vi "Set BackColor.vi"(8 "error in":errorcluster, 10 "Color":T1, 11 "View in":refnum<class "Cell View.lvclass">) -> (0 "error out":errorcluster, 3 "View out":refnum<class "Cell View.lvclass">)   [LabVIEW 2023, in "SourceGrid.lvlib" / "Cell View.lvclass"]
uses:
  Cell View.lvclass
  Cell View.lvclass/Cell View.ctl
  D:/git/Sourcegrid-LabVIEW/dll/SourceGrid.dll
  dll/SourceGrid.dll
  Color/Color.lvclass
  System.Drawing.Color.ctl
  SourceGrid.lvlib
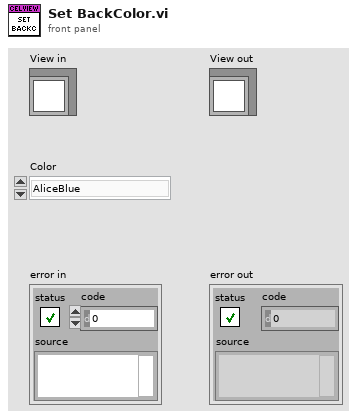
[diagram p1: front panel]
types:
  T1 = typedef "SourceGrid.lvlib/System.Drawing.Color.ctl" = enum16{"AliceBlue", "AntiqueWhite", "Aqua", "Aquamarine", "Azure", "Beige", "Bisque", "Black", "BlanchedAlmond", "Blue", "BlueViolet", "Brown", "BurlyWood", "CadetBlue", "Chartreuse", "Chocolate", "Coral", "CornflowerBlue", "Cornsilk", "Crimson", "Cyan", "DarkBlue", "DarkCyan", "DarkGoldenrod", "DarkGray", "DarkGreen", "DarkKhaki", "DarkMagenta", "DarkOliveGreen", "DarkOrange", "DarkOrchid", "DarkRed", "DarkSalmon", "DarkSeaGreen", "DarkSlateBlue", "DarkSlateGray", "DarkTurquoise", "DarkViolet", "DeepPink", "DeepSkyBlue", "DimGray", "DodgerBlue", "Firebrick", "FloralWhite", "ForestGreen", "Fuchsia", "Gainsboro", "GhostWhite", "Gold", "Goldenrod", "Gray", "Green", "GreenYellow", "Honeydew", "HotPink", "IndianRed", "Indigo", "Ivory", "Khaki", "Lavender", "LavenderBlush", "LawnGreen", "LemonChiffon", "LightBlue", "LightCoral", "LightCyan", "LightGoldenrodYellow", "LightGray", "LightGreen", "LightPink", "LightSalmon", "LightSeaGreen", "LightSkyBlue", "LightSlateGray", "LightSteelBlue", "LightYellow", "Lime", "LimeGreen", "Linen", "Magenta", "Maroon", "MediumAquamarine", "MediumBlue", "MediumOrchid", "MediumPurple", "MediumSeaGreen", "MediumSlateBlue", "MediumSpringGreen", "MediumTurquoise", "MediumVioletRed", "MidnightBlue", "MintCream", "MistyRose", "Moccasin", "NavajoWhite", "Navy", "OldLace", "Olive", "OliveDrab", "Orange", "OrangeRed", "Orchid", "PaleGoldenrod", "PaleGreen", "PaleTurquoise", "PaleVioletRed", "PapayaWhip", "PeachPuff", "Peru", "Pink", "Plum", "PowderBlue", "Purple", "Red", "RosyBrown", "RoyalBlue", "SaddleBrown", "Salmon", "SandyBrown", "SeaGreen", "SeaShell", "Sienna", "Silver", "SkyBlue", "SlateBlue", "SlateGray", "Snow", "SpringGreen", "SteelBlue", "Tan", "Teal", "Thistle", "Tomato", "Transparent", "Turquoise", "Violet", "Wheat", "White", "WhiteSmoke", "Yellow"}
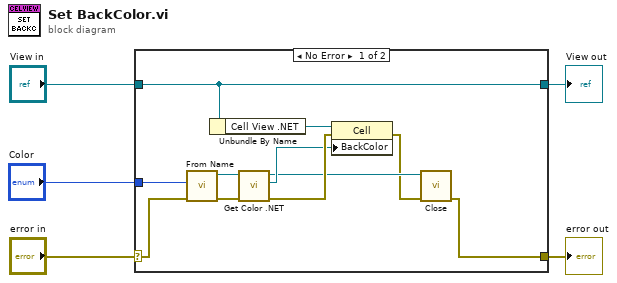
[diagram p0: block diagram]
diagram:
  n1 = case shown="No Error" "error in" {
    selector: "error in" -> [w12 w16]
    tunnel: [w6 w16] -> w4
    tunnel: [w14 w17] -> w2
    tunnel: "View in" -> [w14 w17]
    tunnel: "Color" -> [w13 _]
    frame No Error {
      n2 = call "From Name.vi"("error in"=w12, "Color"=w13) -> ("error out"=w11:errorcluster, "Color out"=w10:refnum<class "Color.lvclass">)  [unwired: 8 in]
      n3 = Unbundle By Name(w14) -> ("Cell View .NET"=w15:refnum<k24>)
      n4 = call "Get Color .NET.vi"("Color in"=w10) -> ("Color .NET"=w9:refnum<k24>, "Color out"=w8:refnum<class "Color.lvclass">)  [unwired: 9 in]
      n5 = property class="Cell"(reference=w15, error in=w11, "BackColor"=w9) -> (error out=w7:errorcluster)  [unwired: 1 out]
      n6 = call-dynamic "Close.vi"("error in"=w7, "Color in"=w8) -> ("error out"=w6:errorcluster)  [unwired: 8 in, 1 out]
    }
    frame Error {
    }
  }
  "error out" <- w4
  "View out" <- w2
